vi "Create.vi"(8 "error in (no error)":errorcluster, 10 "3D Picture":refnum<vi>, 11 "XRay Scene in":refnum<class "XRay Scene.lvclass">) -> (0 "error out":errorcluster, 3 "XRay Scene out":refnum<class "XRay Scene.lvclass">)   [LabVIEW 2026, in "XRay Scene.lvclass"]
uses:
  XRay Scene.lvclass
  XRay Scene.lvclass/XRay Scene.ctl
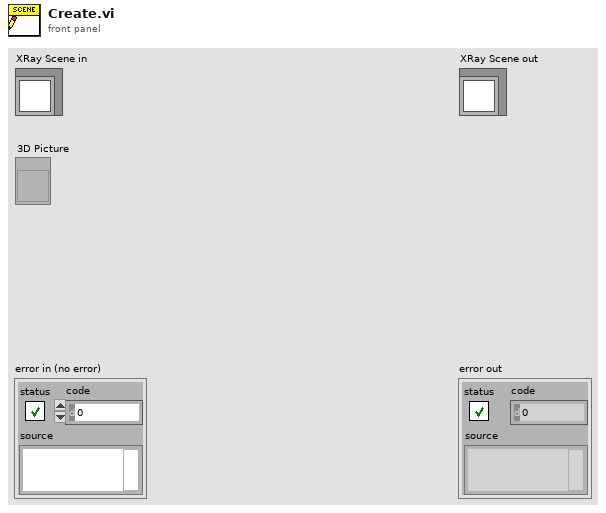
[diagram p1: front panel]
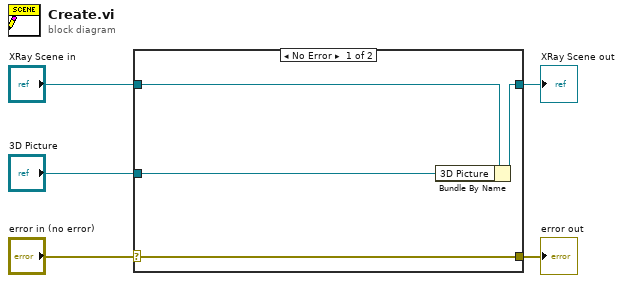
[diagram p0: block diagram]
diagram:
  n1 = case shown="No Error" "error in (no error)" {
    selector: "error in (no error)" -> [w9 w10]
    tunnel: [w9 w10] -> w4
    tunnel: [w7 w11] -> w2
    tunnel: "XRay Scene in" -> [w8 w11]
    tunnel: "3D Picture" -> [w6 _]
    frame No Error {
      n2 = Bundle By Name(cluster=w8, "3D Picture"=w6) -> (w7:refnum<class "XRay Scene.lvclass">)
    }
    frame Error {
    }
  }
  "error out" <- w4
  "XRay Scene out" <- w2
